vi "DT_Post.vi"(9 "output option":T1 items=["Triangle", "Adj Triangle", "Segment"], 10 "Points":cluster{"x":dbl, "y":dbl, "index":i32}[](array[cluster]), 11 "Triangles In":i32[][](array[numeric])) -> (3 "Triangles Out":i32[][](array[numeric]))   [LabVIEW 2020, in "NI_AAL_Geometry.lvlib"]
uses:
  <vilib>/Analysis/NI_AAL_Geometry.lvlib
  <vilib>/Analysis/geometry.llb/DT_Output Option.ctl
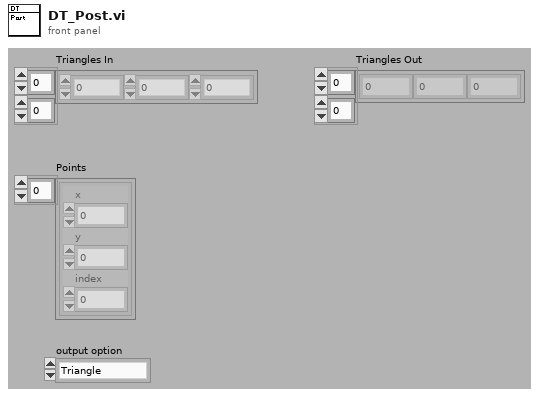
[diagram p1: front panel]
types:
  T1 = typedef "NI_AAL_Geometry.lvlib/DT_Output Option.ctl" = i32
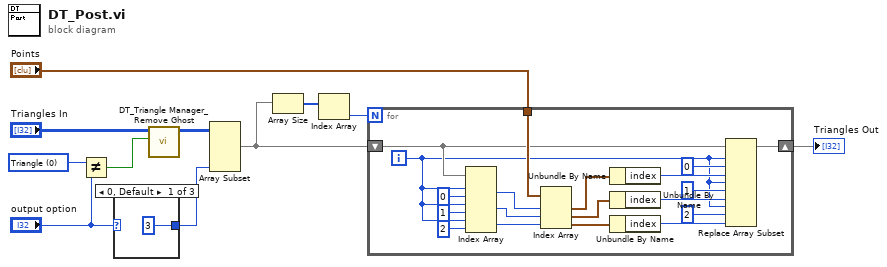
[diagram p0: block diagram]
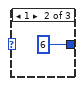
[diagram p2: hidden frame]
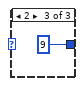
[diagram p3: hidden frame]
diagram:
  w4 = T1 0 items=["Triangle", "Adj Triangle", "Segment"] ("x")
  n1 = Not Equal?(x=w4, y="output option") -> (x != y?=w6:bool)
  n2 = case shown="0, Default" "output option" {
    tunnel: [3 6 9] -> w7
    frame 0, Default {
    }
    frame 1 {
    }
    frame 2 {
    }
  }
  n3 = call <vilib>:"DT_Triangle Manager_Remove Ghost.vi"("update adj tri?"=w6, "Triangles In"="Triangles In") -> ("Triangles Out"=w8:i32[][])  [unwired: 9 out]
  n4 = Array Subset(array=w8, length (col)=w7) -> (w3:i32[][])  [unwired: 3 in]
  n5 = Array Size(array=w3) -> (size(s)=w2:i32[])
  n6 = Index Array(array=w2) -> (element=w1:i32)  [unwired: 1 in]
  n7 = for {
    N: w1 -> [_]
    tunnel: "Points" -> [w33]
    shift-right: [w32] -> w10
    shift-left: w3 -> [w19]
    i -> [w18]
    n8 = Index Array(array=w19, index (row) #1=w18, index (col) #1=0 ("disabled index (col)"), index (row) #2=w18, index (col) #2=1 ("disabled index (col)"), index (row) #3=w18, index (col) #3=2 ("disabled index (col)")) -> (element #1=w22:i32, element #2=w21:i32, element #3=w20:i32)
    n9 = Index Array(array=w33, index #1=w22, index #2=w21, index #3=w20) -> (element #1=w31:cluster{"x":dbl, "y":dbl, "index":i32}, element #2=w30:cluster{"x":dbl, "y":dbl, "index":i32}, element #3=w29:cluster{"x":dbl, "y":dbl, "index":i32})
    n10 = Unbundle By Name(w31) -> ("index"=w27:i32)
    n11 = Unbundle By Name(w30) -> ("index"=w23:i32)
    n12 = Unbundle By Name(w29) -> ("index"=w26:i32)
    n13 = Replace Array Subset(array=w19, new element #1=w27, index (row) #1=w18, index (col) #1=0 ("disabled index (col)"), new element #2=w23, index (row) #2=w18, index (col) #2=1 ("disabled index (col)"), new element #3=w26, index (row) #3=w18, index (col) #3=2 ("disabled index (col)")) -> (w32:i32[][])
  }
  "Triangles Out" <- w10
